vi "setup.vi"(8 "error in (no error)":errorcluster, 11 "Analog_Output in":refnum<class "Analog_Output.lvclass">) -> (0 "error out":errorcluster, 3 "Analog_Output out":refnum<class "Analog_Output.lvclass">)   [LabVIEW 2013, in "Analog_Output.lvclass"]
uses:
  Analog_Output.lvclass
  Analog_Output.lvclass/Analog_Output.ctl
  Globals.vi
  <vilib>/DAQmx/create/channels.llb/DAQmx Create Channel (AO-Voltage-Basic).vi
  <vilib>/DAQmx/configure/timing.llb/DAQmx Timing (Sample Clock).vi
  <vilib>/DAQmx/configure/trigger.llb/DAQmx Start Trigger (Digital Edge).vi
  <vilib>/DAQmx/configure/events/hardwareSignals.llb/DAQmx Export Signal (Most Signals).vi
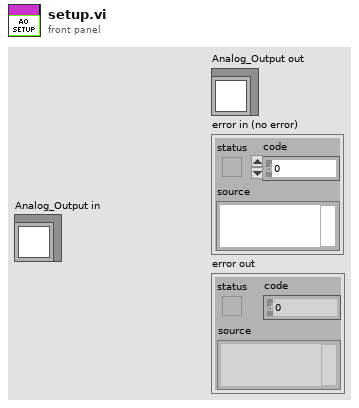
[diagram p1: front panel]
types:
  T1 = typedef "Analog_Output.lvclass/AO_settings.ctl" = cluster{"Enable Analog Out?":bool, "Physical Channel":tag, "Minimum Value":dbl, "Maximum Value":dbl, "Samples per second":dbl, "Start Trigger":cluster{"Wait for start trigger?":bool, "source":tag, "edge":i32}, "Analog Output Waveforms (channel, time)":dbl[][], "Export trigger":cluster{"Export Start Trigger?":bool, "output terminal":tag}, "External Clock":cluster{"Use external clock?":bool, "source":tag, "max expected clock rate":dbl}}
  T2 = cluster{"Wait for start trigger?":bool, "source":tag, "edge":i32}
  T3 = cluster{"Export Start Trigger?":bool, "output terminal":tag}
  T4 = cluster{"Use external clock?":bool, "source":tag, "max expected clock rate":dbl}
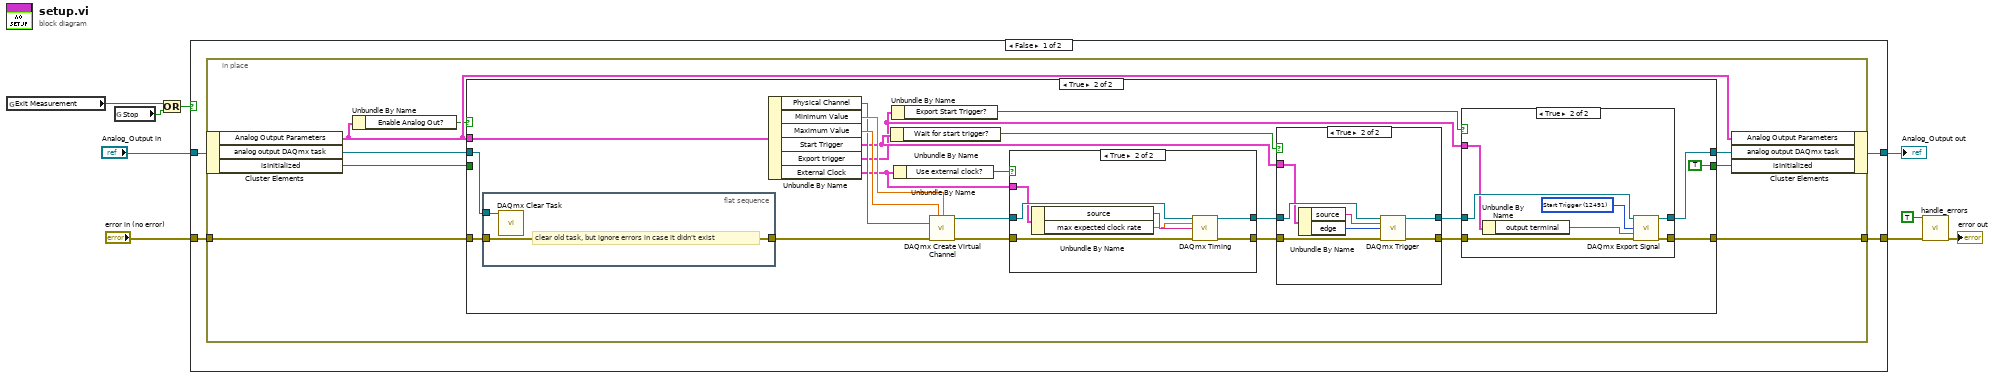
[diagram p0: block diagram]
diagram:
  n1 = global read "Globals.vi" "Exit Measurement"() -> (w8:bool)
  n2 = global read "Globals.vi" "Stop"() -> (w7:bool)
  n3 = Or(x=w8, y=w7) -> (x .or. y?=w5:bool)
  n4 = case shown="False" w5 {
    tunnel: [w12 w77] -> w9
    tunnel: "Analog_Output in" -> [w13 w77]
    tunnel: "error in (no error)" -> [w11 w76]
    tunnel: [w10 w76] -> w2
    frame False {
      n5 = in-place {
        in-place-border: w11 -> [w20]
        in-place-border: [w18] -> w10
        n6 = in-place-cluster #1(w13) -> ("Analog Output Parameters"=w21:T1, "analog output DAQmx task"=w19:refnum<k21>, "isInitialized"=w14:bool)
        n7 = Unbundle By Name(w21) -> ("Enable Analog Out?"=w15:bool)
        n8 = case shown="True" w15 {
          tunnel: w20 -> [w24 w32]
          tunnel: [w24 w39] -> w18
          tunnel: [w23 w38] -> w16
          tunnel: w21 -> [_ w46]
          tunnel: w19 -> [w23 w33]
          tunnel: [w22 TRUE ("isInitialized")] -> w17
          tunnel: w14 -> [w22 _]
          frame False {
          }
          frame True {
            n9 = flat-sequence {
              tunnel: w33 -> [w57]
              tunnel: w32 -> [w56]
              tunnel: [w56] -> w31
              frame #0 {
                # "clear old task, but ignore errors in case it didn't exist"
                n10 = call <vilib>:"DAQmx Clear Task.vi"("task in"=w57) -> ()  [unwired: 14 in, 1 out]
              }
            }
            n11 = Unbundle By Name(w46) -> ("Physical Channel"=w43:tag, "Minimum Value"=w45:dbl, "Maximum Value"=w44:dbl, "Start Trigger"=w42:T2, "Export trigger"=w34:T3, "External Clock"=w25:T4)
            n12 = Unbundle By Name(w42) -> ("Wait for start trigger?"=w41:bool)
            n13 = Unbundle By Name(w34) -> ("Export Start Trigger?"=w35:bool)
            n14 = Unbundle By Name(w25) -> ("Use external clock?"=w26:bool)
            n15 = call-poly <vilib>:"DAQmx Create Virtual Channel.vi"("maximum value"=w44, "minimum value"=w45, "physical channels"=w43, "error in"=w31) -> ("task out"=w30:refnum<k21>, "error out"=w28:errorcluster)  [unwired: 10 in]
            n16 = case shown="True" w26 {
              tunnel: w30 -> [w48 w55]
              tunnel: [w48 w54] -> w29
              tunnel: w28 -> [w47 w53]
              tunnel: [w47 w52] -> w27
              tunnel: w25 -> [_ w51]
              frame False {
              }
              frame True {
                n17 = Unbundle By Name(w51) -> ("source"=w50:tag, "max expected clock rate"=w49:dbl)
                n18 = call-poly <vilib>:"DAQmx Timing.vi"("task/channels in"=w55, "rate"=w49, "source"=w50, "error in"=w53) -> ("task out"=w54:refnum<k21>, "error out"=w52:errorcluster)  [unwired: 10 in]
              }
            }
            n19 = case shown="True" w41 {
              tunnel: [w68 w75] -> w40
              tunnel: [w67 w74] -> w37
              tunnel: w29 -> [w67 w73]
              tunnel: w27 -> [w68 w72]
              tunnel: w42 -> [_ w71]
              frame False {
              }
              frame True {
                n20 = Unbundle By Name(w71) -> ("source"=w70:tag, "edge"=w69:i32)
                n21 = call-poly <vilib>:"DAQmx Trigger.vi"("task/channels in"=w73, "source"=w70, "edge"=w69, "error in"=w72) -> ("task out"=w74:refnum<k21>, "error out"=w75:errorcluster)  [unwired: 10 in]
              }
            }
            n22 = case shown="True" w35 {
              tunnel: w40 -> [w58 w65]
              tunnel: [w58 w64] -> w39
              tunnel: [w59 w63] -> w38
              tunnel: w37 -> [w59 w62]
              tunnel: w34 -> [_ w61]
              frame False {
              }
              frame True {
                w66 = 12491 items=["AI Convert Clock"=12484, "10MHz Reference Clock"=12536, "20MHz Timebase Clock"=12486, "Sample Clock"=12487, "Advance Trigger"=12488, "Reference Trigger"=12490, "Start Trigger"=12491, "Advance Complete Event"=12492, "AI Hold Complete Event"=12493, "Counter Output Event"=12494, "Change Detection Event"=12511, "Watchdog Timer Expired Event"=12512] ("signal")
                n23 = Unbundle By Name(w61) -> ("output terminal"=w60:tag)
                n24 = call-poly <vilib>:"DAQmx Export Signal.vi"("task/channels in"=w62, "signal"=w66, "output terminal"=w60, "error in"=w65) -> ("task out"=w63:refnum<k21>, "error out"=w64:errorcluster)  [unwired: 10 in]
              }
            }
          }
        }
        n25 = in-place-cluster #1("Analog Output Parameters"=w21, "analog output DAQmx task"=w16, "isInitialized"=w17) -> (w12:refnum<class "Analog_Output.lvclass">)
      }
    }
    frame True {
    }
  }
  "Analog_Output out" <- w9
  n26 = call "handle_errors.vi"("Exit Operation"=TRUE, "error in (no error)"=w2) -> ("error out"=→"error out":errorcluster)  [unwired: 13 in]
